vi "Database.Handler.vi"() -> ()   [LabVIEW 2016]
uses:
  Database.Handler.Action.ctl
  Database.Handler.Data.ctl
  Database.Handler.Data.Sets.ctl
  Database.Handler.Data.Status.ctl
  Tools/EventLog/EventLog.EventSource.ctl
  Tools/CitTemplate/citTemplate.errData.ctl
  Database.Global.vi
panel:
  out "error.action":string
  out "error":errorcluster
  out "_loop":i32(ring)=4
  out "action":T1=enum."--- DB.Handler ---"
  out "Data":T2
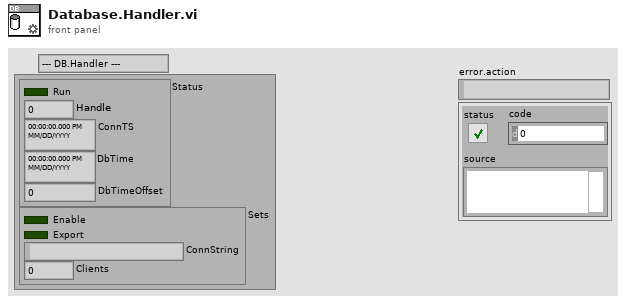
[diagram p1: front panel]
types:
  T1 = typedef "Database.Handler.Action.ctl" = enum32{"idle", "constructor", "destructor", "--- DB.Handler ---", "Setup", "Reconnect", "ReconnectAll", "ReconnectOne", "ExportData"}
  T2 = typedef "Database.Handler.Data.ctl" = cluster{"Status":T3, "Sets":T4}
  T3 = typedef "Database.Handler.Data.Status.ctl" = cluster{"Run":bool, "Handle":i32, "ConnTS":timestamp, "DbTime":timestamp, "DbTimeOffset":dbl}
  T4 = typedef "Database.Handler.Data.Sets.ctl" = cluster{"Enable":bool, "Export":bool, "ConnString":string, "Clients":i32}
  T5 = typedef "citTemplate.errData.ctl" = cluster{"ts":timestamp, "src":T6, "instance":i32, "action":string, "error":errorcluster, "unconfirmed":bool}
  T6 = typedef "EventLog.EventSource.ctl" = enum16{"All", "Gui", "Cache", "PLC1", "PLC2", "PLC3", "DB", "DB01", "DB02", "DB03", "DB04", "DB05", "DB06", "DB07", "DB08", "DB09", "DB10", "DB11", "DB12", "DB13", "DB14", "DB15", "DB16"}
  T7 = typedef "citTemplate.notifierHandle.ctl" = refnum<notifier>
  T8 = typedef "Database.Data.Sets.ctl" = cluster{"Enable":bool, "ConnString":string, "SystemName":string, "Process.Begin":bool, "Process.End":bool}
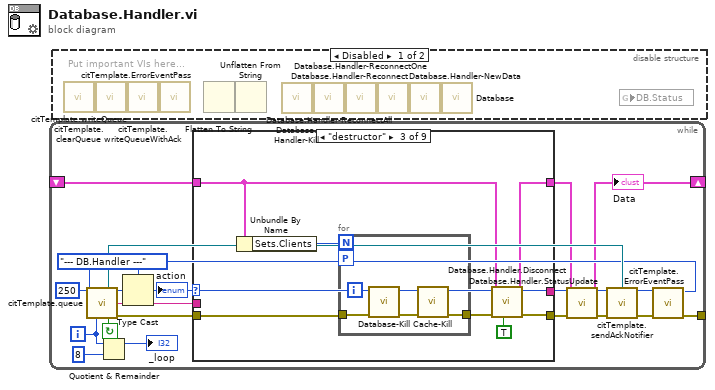
[diagram p0: block diagram]
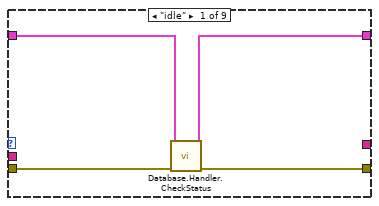
[diagram p2: hidden frame]
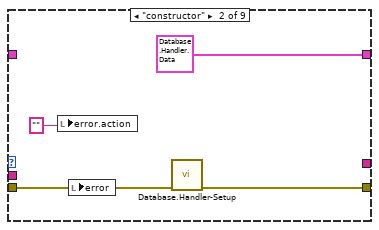
[diagram p3: hidden frame]
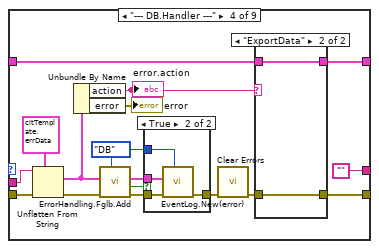
[diagram p4: hidden frame]
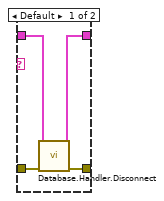
[diagram p5: hidden frame]
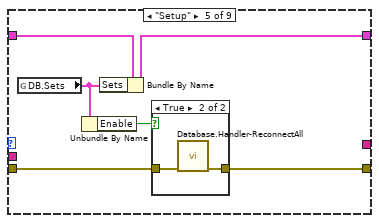
[diagram p7: hidden frame]
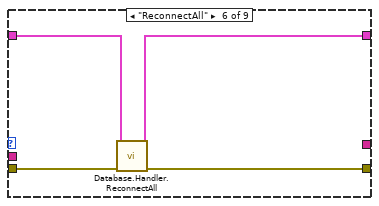
[diagram p9: hidden frame]
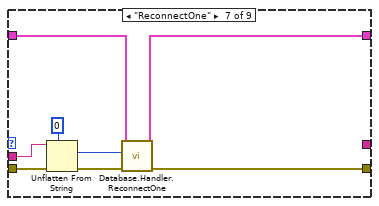
[diagram p10: hidden frame]
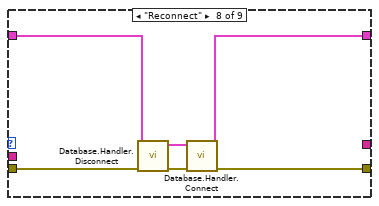
[diagram p11: hidden frame]
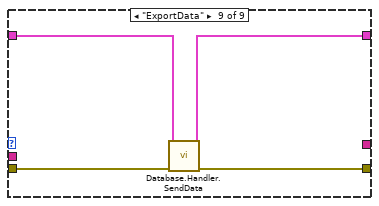
[diagram p12: hidden frame]
diagram:
  n1 = while {
    tunnel: [w12] -> _
    shift-right: [w2] -> _
    shift-left: _ -> [w1]
    i -> [w13]
    stop <- w15 continue-if-true
    w6 = Database.Handler.Action."--- DB.Handler ---" ("Action")
    n2 = call "citTemplate.queue.vi"("ms timeout (250 ms)"=250, "event enum"=w6, "iteration (-1)"=w13) -> ("notifierHandle out"=w7:T7, "event out"=w18:u32, "(flatten) data out"=w17:string, "continue"=w15:bool, "error out"=w16:errorcluster)  [unwired: 8 in]
    n3 = Quotient & Remainder(x=w13, y=8) -> (x-y*floor(x/y)=→"_loop":i32)  [unwired: 1 out]
    n4 = Type Cast(type=w6, x=w18) -> (*(type *) &x=w11:T1)
    "action" <- w11
    n5 = case shown="\"destructor\"" w11 {
      tunnel: w17 -> [_ _ _ w47 _ _ w84 _ _]
      tunnel: w16 -> [w22 w24 w33 w53 w70 w76 w85 w89 w92]
      tunnel: [w21 w23 w32 w49 w66 w77 w79 w87 w94] -> w5
      tunnel: [w20 T2 {"Status"={"Run"=FALSE, "Handle"=0, "ConnTS"=timestamp(0 s since 1904-01-01), "DbTime"=timestamp(0 s since 1904-01-01), "DbTimeOffset"=0.0}, "Sets"={"Enable"=FALSE, "Export"=FALSE, "ConnString"="", "Clients"=0}} ("Data") w30 w50 w69 w75 w78 w86 w95] -> w3
      tunnel: [_ _ _ "" _ _ _ _ _] -> w8
      tunnel: w1 -> [w19 _ w31 w51 w68 w74 w81 w88 w93]
      frame "idle" {
        n6 = call "Database.Handler.CheckStatus.vi"("error in (no error)"=w22, "Data in"=w19) -> ("error out"=w21:errorcluster, "Data out"=w20:T2)  [unwired: 8 in]
      }
      frame "constructor" {
        n7 = local write "error.action"("" ("error.action")) -> ()
        n8 = local write "error"(w24) -> ()
        n9 = call "Database.Handler-Setup.vi"("error in"=w24) -> ("error out"=w23:errorcluster)  [unwired: 10 in]
      }
      frame "destructor" {
        n10 = Unbundle By Name(w31) -> ("Sets.Clients"=w27:i32)
        n11 = for {
          N: w27 -> [_]
          tunnel: w33 -> [w37]
          tunnel: [w34] -> w29
          workers-P: _ -> [_]
          i -> [w36]
          n12 = call "Database-Kill.vi"("error in"=w37, "Idx"=w36) -> ("error out"=w35:errorcluster)  [unwired: 9 in]
          n13 = call "Cache-Kill.vi"("error in"=w35, "Idx"=w36) -> ("error out"=w34:errorcluster)  [unwired: 9 in]
        }
        n14 = call "Database.Handler.Disconnect.vi"("ReInitDLL (F)"=TRUE, "error in (no error)"=w29, "Data in"=w31) -> ("error out"=w32:errorcluster, "Data out"=w30:T2)  [unwired: 7 in]
      }
      frame "--- DB.Handler ---" {
        w38 = EventLog.EventSource."DB" ("Event source")
        n15 = Unflatten From String(type=T5 {"ts"=timestamp(0 s since 1904-01-01), "src"=enum."All", "instance"=0, "action"="", "error"={"status"=FALSE, "code"=0, "source"=""}, "unconfirmed"=FALSE} ("ErrData"), binary string=w47, error in (no error)=w53) -> (value=w40:T5, error out=w43:errorcluster)  [unwired: 3 out]
        n16 = Unbundle By Name(w40) -> ("action"=w39:string, "error"=→"error":errorcluster)
        "error.action" <- w39
        n17 = call "ErrorHandling.Fglb.Add.vi"("Event source"=w38, "error in (no error)"=w43, "Error in"=w40) -> ("error out"=w45:errorcluster, "changed?"=w44:bool)  [unwired: 7 in]
        n18 = case shown="True" w44 {
          tunnel: [w60 w64] -> w42
          tunnel: w40 -> [_ w63]
          tunnel: w45 -> [w60 w62]
          tunnel: w38 -> [_ w61]
          frame False {
          }
          frame True {
            n19 = call "EventLog.New(error).vi"("Source (All)"=w61, "error in"=w62, "ErrData"=w63) -> ("error out"=w64:errorcluster)  [unwired: 8 in]
          }
        }
        n20 = call <vilib>:"Clear Errors.vi"("error in (no error)"=w42) -> ("error out"=w48:errorcluster)  [unwired: 5 in, 1 out]
        n21 = case shown="\"ExportData\"" w39 {
          tunnel: w51 -> [w57 w58]
          tunnel: [w56 w58] -> w50
          tunnel: [w55 w59] -> w49
          tunnel: w48 -> [w54 w59]
          frame Default {
            n22 = call "Database.Handler.Disconnect.vi"("error in (no error)"=w54, "Data in"=w57) -> ("error out"=w55:errorcluster, "Data out"=w56:T2)  [unwired: 8 in]
          }
          frame "ExportData" {
          }
        }
      }
      frame "Setup" {
        n23 = global read "Database.Global.vi" "DB.Sets"() -> (w65:T8)
        n24 = Unbundle By Name(w65) -> ("Enable"=w67:bool)
        n25 = Bundle By Name(cluster=w68, "Sets"=w65) -> (w69:T2)
        n26 = case shown="True" w67 {
          tunnel: w70 -> [w71 w73]
          tunnel: [w71 w72] -> w66
          frame False {
          }
          frame True {
            n27 = call "Database.Handler-ReconnectAll.vi"("error in"=w73) -> ("error out"=w72:errorcluster)  [unwired: 10 in]
          }
        }
      }
      frame "ReconnectAll" {
        n28 = call "Database.Handler.ReconnectAll.vi"("error in (no error)"=w76, "Data in"=w74) -> ("error out"=w77:errorcluster, "Data out"=w75:T2)  [unwired: 8 in]
      }
      frame "ReconnectOne" {
        n29 = Unflatten From String(type=0 ("Sets.Clients"), binary string=w84, error in (no error)=w85) -> (value=w80:i32, error out=w82:errorcluster)  [unwired: 2 in, 1 out]
        n30 = call "Database.Handler.ReconnectOne.vi"("error in (no error)"=w82, "Idx"=w80, "Data in"=w81) -> ("error out"=w79:errorcluster, "Data out"=w78:T2)  [unwired: 7 in]
      }
      frame "Reconnect" {
        n31 = call "Database.Handler.Disconnect.vi"("error in (no error)"=w89, "Data in"=w88) -> ("error out"=w90:errorcluster, "Data out"=w91:T2)  [unwired: 8 in]
        n32 = call "Database.Handler.Connect.vi"("error in"=w90, "Data in"=w91) -> ("error out"=w87:errorcluster, "Data out"=w86:T2)  [unwired: 8 in]
      }
      frame "ExportData" {
        n33 = call "Database.Handler.SendData.vi"("error in"=w92, "Data in"=w93) -> ("error out"=w94:errorcluster, "Data out"=w95:T2)  [unwired: 8 in]
      }
    }
    n34 = call "Database.Handler.StatusUpdate.vi"("error in (no error)"=w5, "Data in"=w3) -> ("error out"=w4:errorcluster, "Data out"=w2:T2)  [unwired: 8 in]
    "Data" <- w2
    n35 = call "citTemplate.sendAckNotifier.vi"("notification data"=w8, "notifierHandle in"=w7, "error in"=w4) -> ()  [unwired: 13 in]
    n36 = call "citTemplate.ErrorEventPass.vi"("error in"=w4, "action of error"=w11, "event in"=w6) -> ("error out"=w12:errorcluster)  [unwired: 8 in]
  }
  n37 = disable-structure shown="Disabled" {
    frame Disabled {
      # "Put important VIs here..."
      n38 = call "citTemplate.clearQueue.vi"() -> ()  [unwired: 14 in, 2 out]
      n39 = call "citTemplate.writeQueue.vi"() -> ()  [unwired: 15 in, 1 out]
      n40 = call "citTemplate.writeQueueWithAck.vi"() -> ()  [unwired: 13 in, 3 out]
      n41 = call "citTemplate.ErrorEventPass.vi"() -> ()  [unwired: 11 in, 1 out]
      n42 = Flatten To String() -> ()  [unwired: 4 in, 3 out]
      n43 = Unflatten From String() -> ()  [unwired: 5 in, 3 out]
      n44 = call "Database.Handler-Kill.vi"() -> ()  [unwired: 11 in, 1 out]
      n45 = call "Database.Handler-ReconnectAll.vi"() -> ()  [unwired: 11 in, 1 out]
      n46 = call "Database.Handler-ReconnectOne.vi"() -> ()  [unwired: 11 in, 1 out]
      n47 = call "Database.Handler-Reconnect.vi"() -> ()  [unwired: 11 in, 1 out]
      n48 = call "Database.Handler-NewData.vi"() -> ()  [unwired: 10 in, 2 out]
      n49 = call "Database.vi"() -> ()  [unwired: 12 in]
      n50 = global read "Database.Global.vi" "DB.Status"() -> ()  [unwired: 1 in]
    }
    frame Enabled {
    }
  }
